vi "New plot1_old.vi"() -> (0 "Closed w":bool)   [LabVIEW 2021]
uses:
  <vilib>/Analysis/NI_AALBase.lvlib
  <vilib>/gmath/NI_Gmath.lvlib
  <vilib>/Analysis/1siggen.llb/Ramp Pattern by Samples.vi
panel:
  in  "Tab Control":enum32{"Graph", "Information"}(tab)
  out "Waveform Graph":waveform(dbl)[](graph) caption="Waveform Graph 2"
  in  "Local Mode":enum32{"Resume", "Hold"}(radio)
  in  "Refresh time":u32
  out "Filename":string
  out "Trace name":string
  out "Mode signal_Global":string
  out "Execution:State":T1(ring)
  out "total \nrefresh time":u32
  out "message":string
  in  "Minimizar":bool
  in  "stop":bool
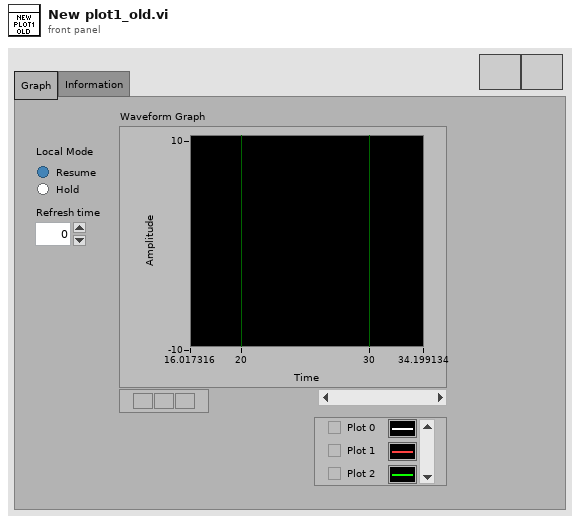
[diagram p1: front panel]
types:
  T1 = enum32{"Bad", "Idle", "Run top level", "Running"}
  T2 = cluster{"plot Names":string[], "Waveforms arrays":waveform(dbl)[], "signals_HW":string[][], "Waveforms arrays csv":waveform(dbl)[], "signals_csv":string[], "Signals_name":string[], "Mode_signal_conf":u8, "Request_plots_array":cluster{string, waveform(dbl)}[], "time out":i32, " global r time":u32}
  T3 = enum32{"Invalid", "Standard", "Closed", "Hidden", "Minimized", "Maximized"}
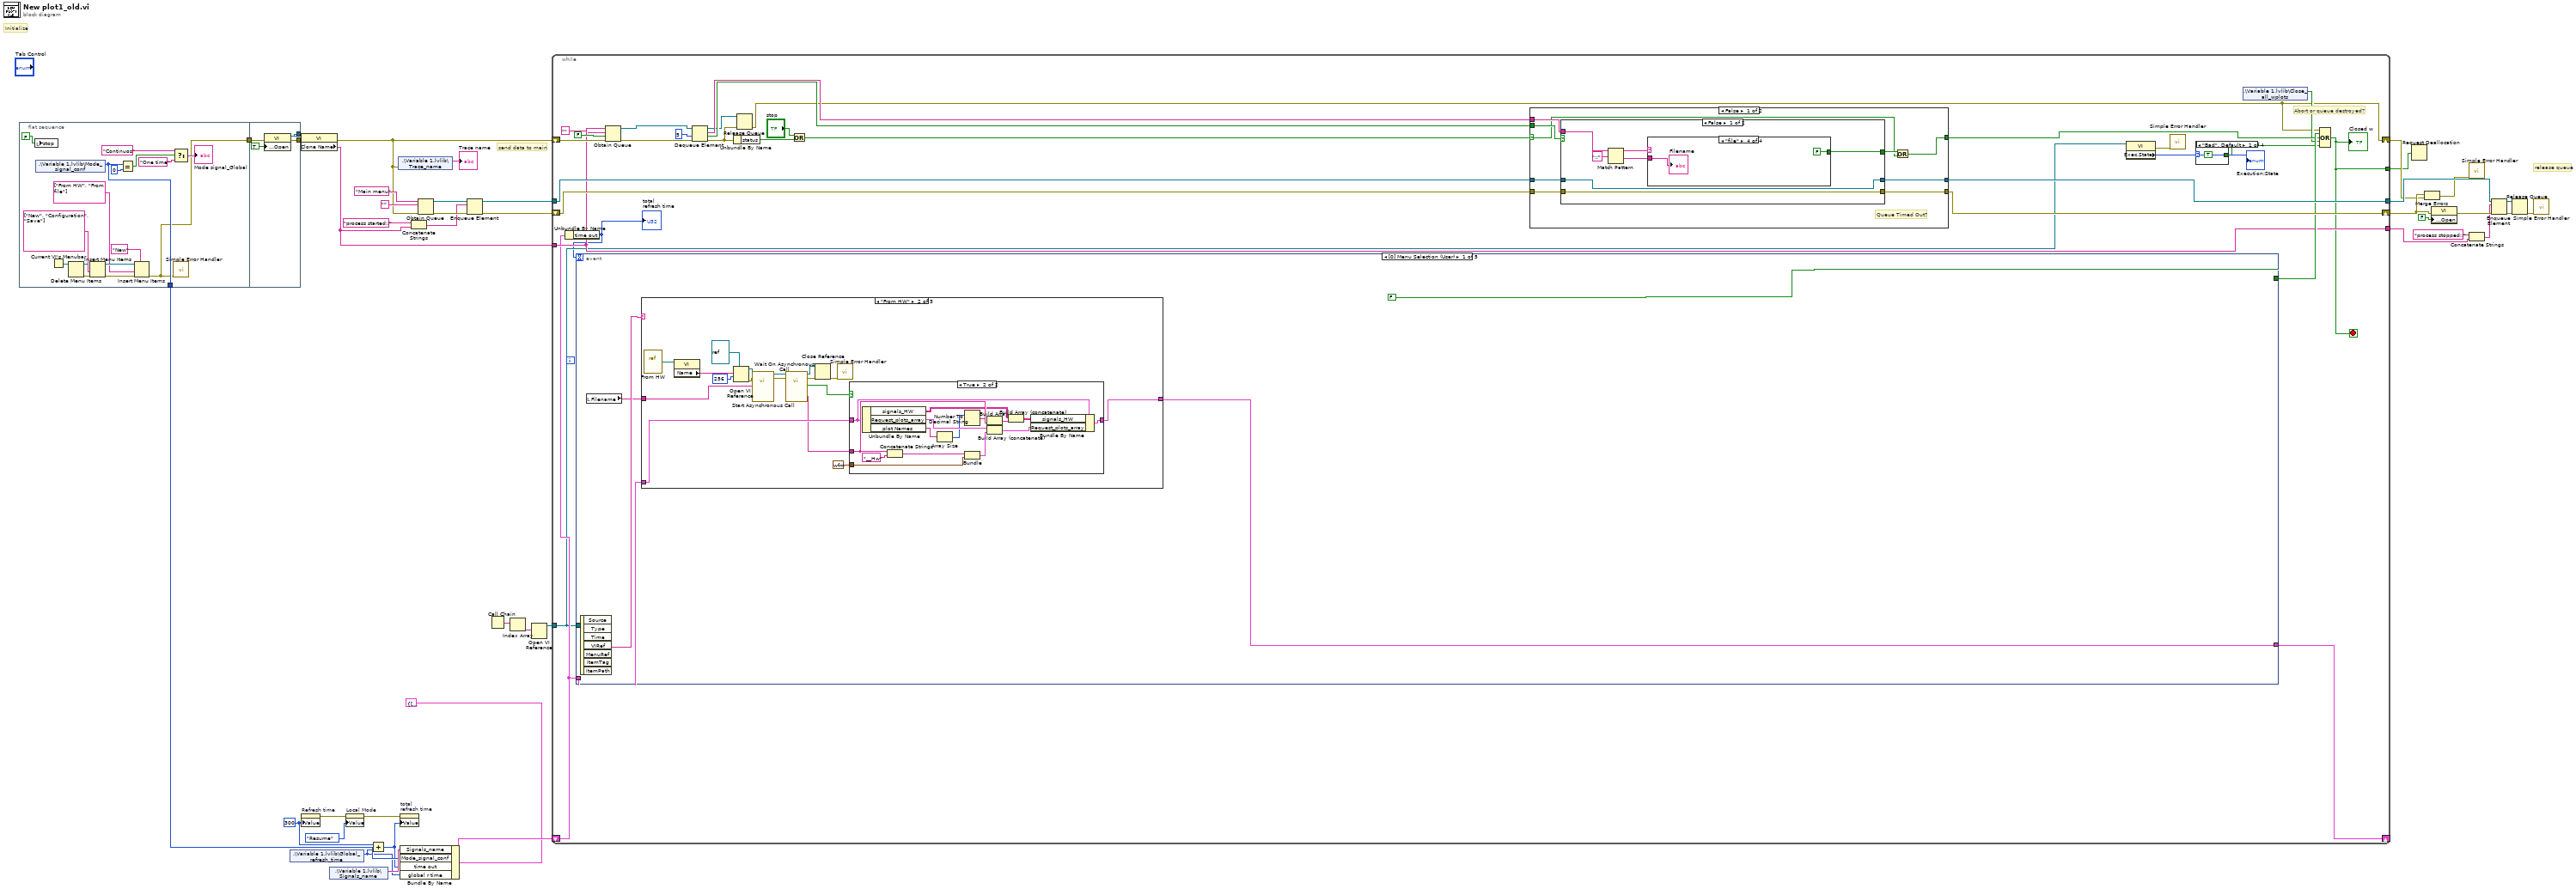
[diagram p0: block diagram]
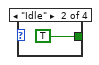
[diagram p2: hidden frame]
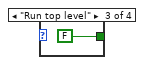
[diagram p3: hidden frame]
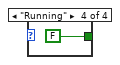
[diagram p4: hidden frame]
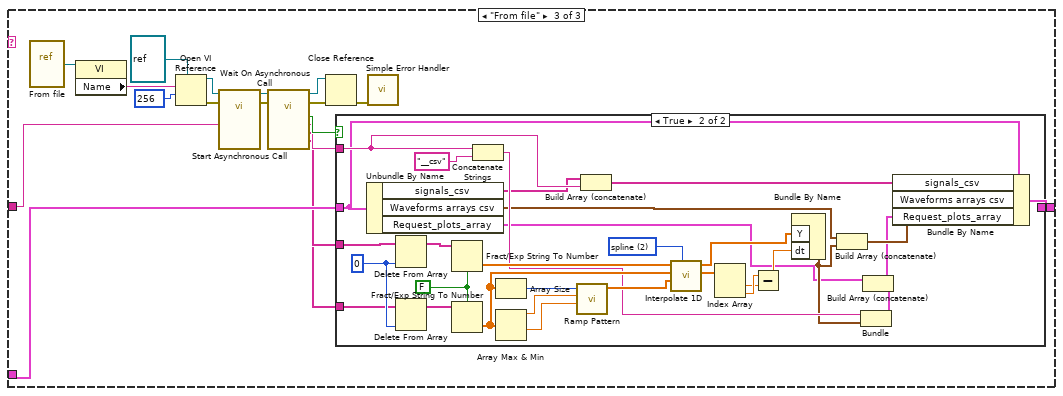
[diagram p7: hidden frame]
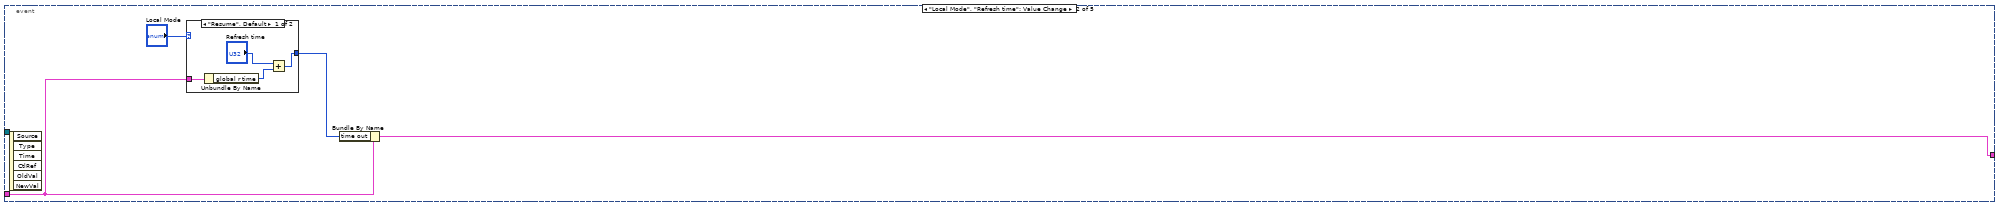
[diagram p9: hidden frame]
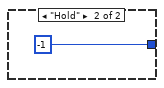
[diagram p10: hidden frame]
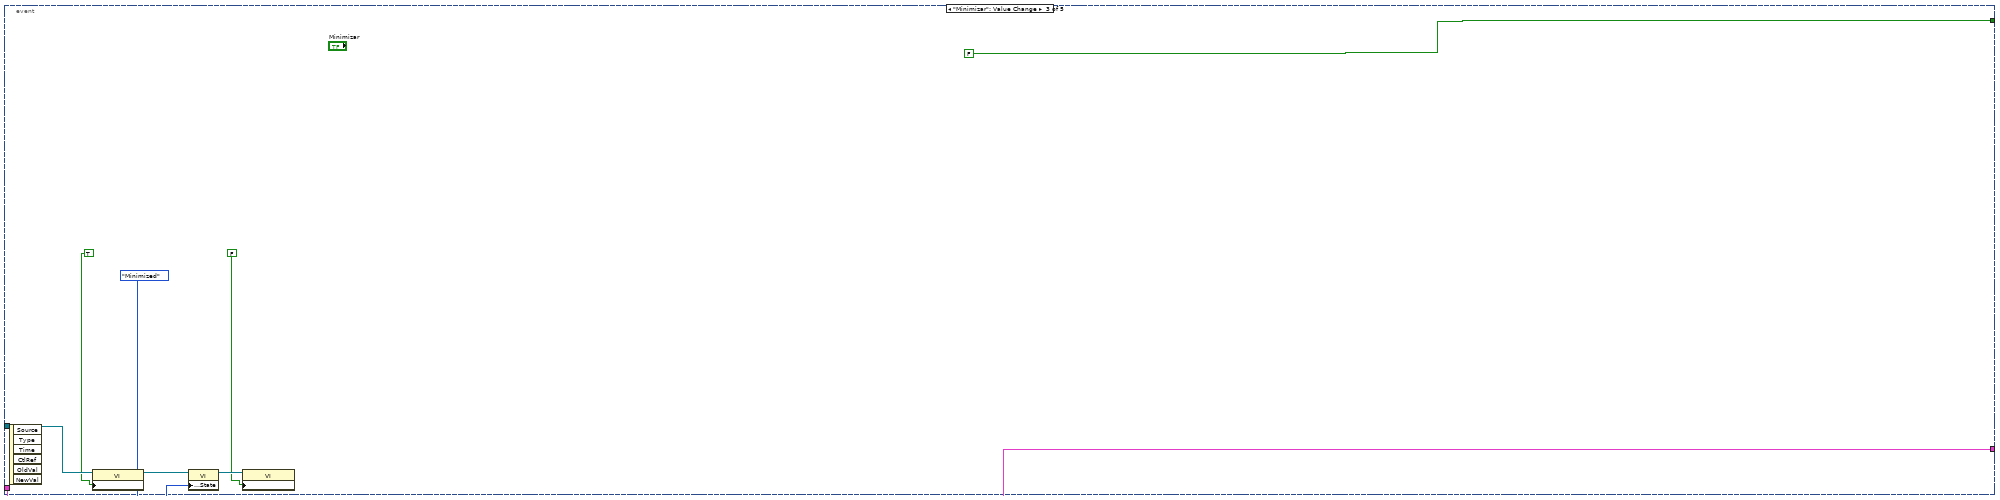
[diagram p11: hidden frame]
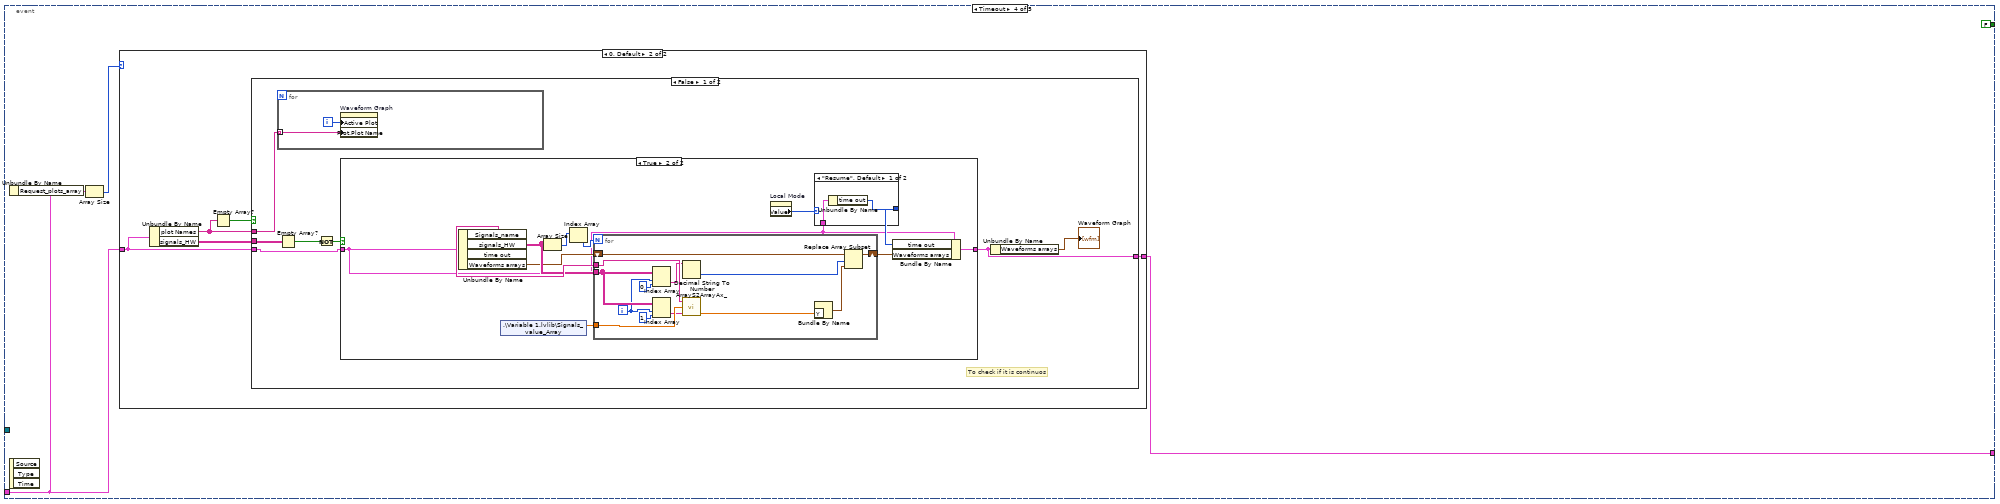
[diagram p12: hidden frame]
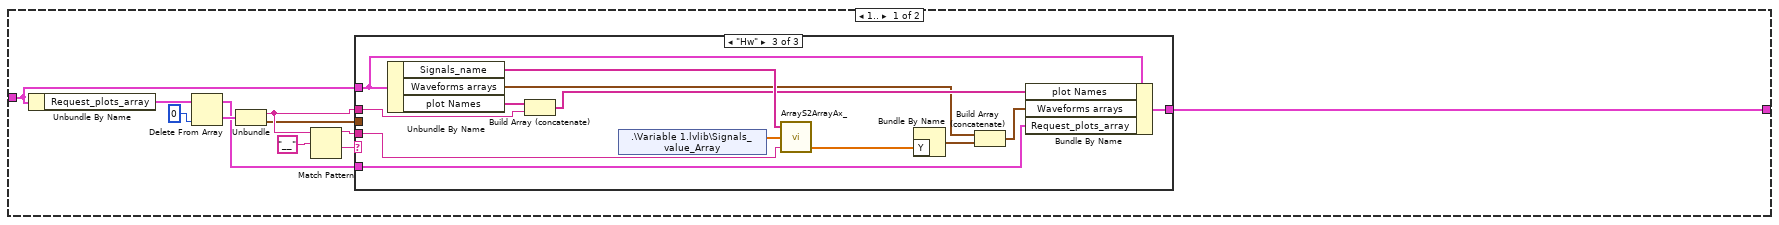
[diagram p13: hidden frame]
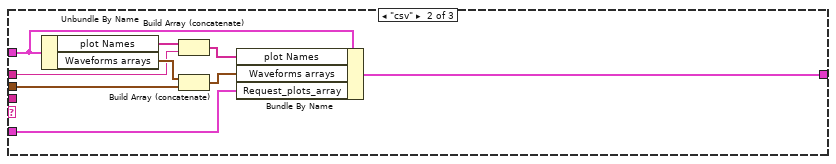
[diagram p15: hidden frame]
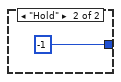
[diagram p17: hidden frame]
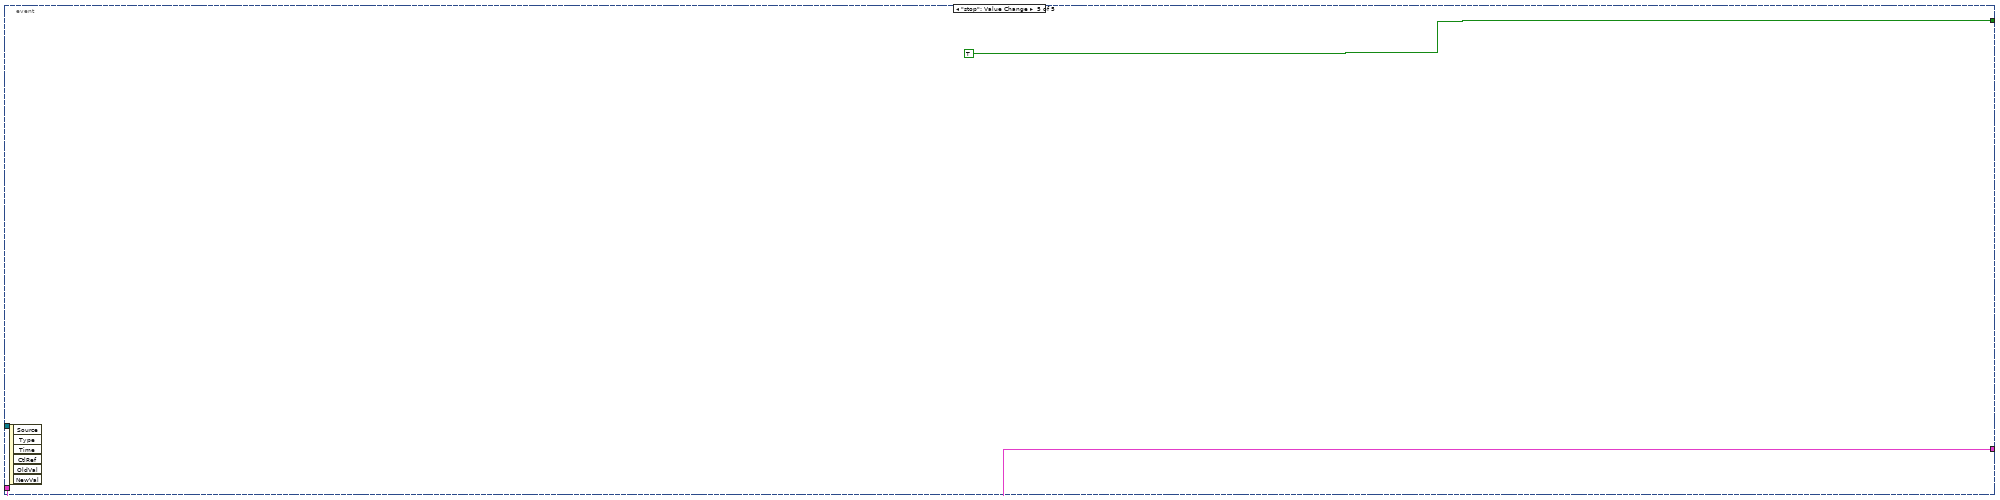
[diagram p19: hidden frame]
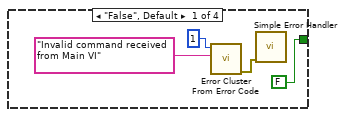
[diagram p20: hidden frame]
diagram:
  w5 = u32 300 ("Refresh time")
  # "Initialize"
  # "send data to main"
  # "release queue"
  n1 = flat-sequence {
    tunnel: [w42] -> w12
    tunnel: [w41] -> w1
    tunnel: [w59] -> w19
    tunnel: [w58] -> w34
    tunnel: w1 -> [w57]
    frame #0 {
      n2 = local write "stop"(FALSE ("stop")) -> ()
      n3 = shared-variable ".\\Variable 1.lvlib\\Mode_signal_conf"() -> (w42:u8)  [unwired: 1 in, 1 out]
      n4 = Current VI's Menubar() -> (w51:refnum<k9>)
      n5 = Delete Menu Items(9:w51) -> (0:w50:errorcluster, 3:w49:refnum<k9>)  [unwired: 3 in]
      n6 = Insert Menu Items(6:w50, 7:string[] ["New", "Configuration", "Save"], 9:w49) -> (0:w56:errorcluster, 3:w55:refnum<k9>)  [unwired: 3 in, 1 out]
      n7 = Equal?(x=w42, y=u8 0) -> (x = y?=w46:bool)
      n8 = Insert Menu Items(5:"New", 6:w56, 7:string[] ["From HW", "From file"], 9:w55) -> (0:w41:errorcluster)  [unwired: 2 in, 2 out]
      n9 = Select(t="Continuos", s=w46, f="One time") -> (s? t:f=→"Mode signal_Global":string)
      n10 = call <vilib>:"Simple Error Handler.vi"("error in (no error)"=w41) -> ()  [unwired: 4 in, 5 out]
    }
    frame #1 {
      n11 = property class="VI"(error in=w57, "Front Panel.Open"=TRUE ("Front Panel Window:Open")) -> (reference out=w59:refnum<vi>, error out=w58:errorcluster)  [unwired: 1 in]
    }
  }
  n12 = shared-variable ".\\Variable 1.lvlib\\Global_refresh_time"() -> (w2:u16)  [unwired: 1 in, 1 out]
  n13 = property class="VI"(reference=w19, error in=w34) -> (error out=w10:errorcluster, "Clone Name"=w11:string)  [unwired: 1 out]
  n14 = property on="Refresh time" class="DigNum (strict)"("Value"=w5) -> (error out=w8:errorcluster)  [unwired: 2 in, 1 out]
  n15 = shared-variable ".\\Variable 1.lvlib\\Signals_name"() -> (w13:string[])  [unwired: 1 in, 1 out]
  n16 = property on="Local Mode" class="RadioBtnsControl (strict)"(error in=w8, "Value"=enum32{"Resume", "Hold"}."Resume" ("Local Mode")) -> (error out=w4:errorcluster)  [unwired: 1 in, 1 out]
  n17 = Add(x=w5, y=w2) -> (x+y=w3:u32)
  n18 = shared-variable ".\\Variable 1.lvlib\\Trace_name"(error in=w10) -> (→"Trace name":string)  [unwired: 1 out]
  n19 = property on="total \nrefresh time" class="DigNum (strict)"(error in=w4, "Value"=w3) -> ()  [unwired: 1 in, 2 out]
  n20 = Bundle By Name(cluster=T2 {"plot Names"=[], "Waveforms arrays"=[], "signals_HW"=[], "Waveforms arrays csv"=[], "signals_csv"=[], "Signals_name"=[], "Mode_signal_conf"=0, "Request_plots_array"=[], "time out"=300, " global r time"=0}, "Signals_name"=w13, "Mode_signal_conf"=w12, "time out"=w3, "global r time"=w2) -> (w14:T2)
  n21 = Concatenate Strings("process started::" ("name (unnamed)"), w11) -> (w35:string)
  n22 = Obtain Queue(name (unnamed)="Main menu", element data type="", error in (no error)=w10) -> (queue out=w37:refnum<queue>, error out=w36:errorcluster)  [unwired: 2 in, 1 out]
  n23 = Enqueue Element(queue=w37, element=w35, error in (no error)=w36) -> (queue out=w33:refnum<queue>, error out=w32:errorcluster)  [unwired: 1 in, 1 out]
  n24 = Call Chain() -> (call chain=w18:string[])
  n25 = Index Array(array=w18) -> (element=w17:string)  [unwired: 1 in]
  n26 = Open VI Reference(vi path=w17) -> (vi reference=w16:refnum<vi>)  [unwired: 5 in, 1 out]
  n27 = while {
    tunnel: w33 -> [w90]
    tunnel: [w88] -> w31
    shift-right: [w87] -> w25
    shift-left: w32 -> [w89]
    shift-right: [w61] -> w24
    shift-left: w10 -> [w78]
    tunnel: [w70] -> w21
    tunnel: w16 -> [w66]
    tunnel: w11 -> [w70]
    shift-right: [w71] -> _
    shift-left: w14 -> [w69]
    tunnel: [w63] -> w7
    stop <- w63 stop-if-true
    # "Abort or queue destroyed?"
    n28 = Unbundle By Name(w69) -> ("time out"=w62:i32)
    "total \nrefresh time" <- w62
    n29 = event shown="[0] Menu Selection (User)" {
      selector: _ -> [_ _ _ _ _]
      dyn-events: _ -> [_ _ _ _ _]
      timeout: w62 -> [_ _ _ _ _]
      tunnel: [FALSE _ FALSE FALSE TRUE] -> w74
      tunnel: w66 -> [_ _ w199 _ _]
      tunnel: [w96 w186 w193 w204 w283] -> w71
      tunnel: w69 -> [w97 w184 w193 w203 w283]
      event Menu Selection (User) {
        n30 = event-data() -> ("ItemTag"=w99:string)  [unwired: 1 in, 6 out]
        n31 = local read "Filename"() -> (w95:string)
        n32 = case shown="\"From HW\"" w99 {
          tunnel: [w100 w112 w144] -> w96
          tunnel: w97 -> [w100 w103 w145]
          tunnel: w95 -> [_ w104 w134]
          frame "False", Default {
          }
          frame "From HW" {
            n33 = vi-ref "From HW.vi"() -> (w113:refnum<vi>)
            n34 = property class="VI"(reference=w113) -> ("Name"=w105:string)  [unwired: 1 in, 2 out]
            n35 = Open VI Reference(type specifier VI Refnum (for type only)=refnum<vi> refnum ("reference"), vi path=w105, options=256) -> (vi reference=w114:refnum<vi>, error out=w117:errorcluster)  [unwired: 3 in]
            n36 = call-by-ref "Start Asynchronous Call"(reference=w114, error in=w117, "Plot window"=w104) -> (reference out=w110:refnum<vi>, error out=w111:errorcluster)  [unwired: 2 in, 3 out]
            n37 = call-by-ref "Wait On Asynchronous Call"(reference=w110, error in=w111) -> (reference out=w109:refnum<vi>, error out=w108:errorcluster, "Y name"=w101:string, "Ready?"=w107:bool)  [unwired: 3 in, 1 out]
            n38 = Close Reference(reference=w109, error in (no error)=w108) -> (error out=w116:errorcluster)
            n39 = call <vilib>:"Simple Error Handler.vi"("error in (no error)"=w116) -> ()  [unwired: 4 in, 5 out]
            n40 = case shown="True" w107 {
              tunnel: w101 -> [_ w132]
              tunnel: [w118 w127] -> w112
              tunnel: w103 -> [w118 w131]
              tunnel: waveform(dbl) {"t0"=timestamp(0 s since 1904-01-01), "dt"=1.0, "Y"=[]} ("Waveform") -> [_ w125]
              frame False {
              }
              frame True {
                n41 = Unbundle By Name(w131) -> ("signals_HW"=w130:string[][], "Request_plots_array"=w124:cluster{string, waveform(dbl)}[], "plot Names"=w121:string[])
                n42 = Concatenate Strings(w132, "__Hw" ("string")) -> (w126:string)
                n43 = Array Size(array=w121) -> (size(s)=w120:i32)
                n44 = Number To Decimal String(number=w120) -> (decimal integer string=w119:string)  [unwired: 1 in]
                n45 = Bundle(w126, "Waveform"=w125) -> (w123:cluster{string, "Waveform":waveform(dbl)})  [unwired: 1 in]
                n46 = Build Array(w119, w132) -> (w129:string[])
                n47 = Build Array (concatenate)(w124, w123) -> (w122:cluster{string, "Waveform":waveform(dbl)}[])
                n48 = Build Array (concatenate)(w130, w129) -> (w128:string[][])
                n49 = Bundle By Name(cluster=w131, "signals_HW"=w128, "Request_plots_array"=w122) -> (w127:T2)
              }
            }
          }
          frame "From file" {
            n50 = vi-ref "From file.vi"() -> (w148:refnum<vi>)
            n51 = property class="VI"(reference=w148) -> ("Name"=w142:string)  [unwired: 1 in, 2 out]
            n52 = Open VI Reference(type specifier VI Refnum (for type only)=refnum<vi> refnum, vi path=w142, options=256) -> (vi reference=w146:refnum<vi>, error out=w151:errorcluster)  [unwired: 3 in]
            n53 = call-by-ref "Start Asynchronous Call"(reference=w146, error in=w151, "Plot window"=w134) -> (reference out=w143:refnum<vi>, error out=w141:errorcluster)  [unwired: 3 in, 4 out]
            n54 = call-by-ref "Wait On Asynchronous Call"(reference=w143, error in=w141) -> (reference out=w136:refnum<vi>, error out=w135:errorcluster, "Y subarray"=w137:string[], "X subarray"=w138:string[], "Curve name"=w139:string, "Ready?"=w140:bool)  [unwired: 4 in]
            n55 = Close Reference(reference=w136, error in (no error)=w135) -> (error out=w150:errorcluster)
            n56 = case shown="True" w140 {
              tunnel: w138 -> [_ w182]
              tunnel: w137 -> [_ w181]
              tunnel: w139 -> [_ w164]
              tunnel: w145 -> [w152 w158]
              tunnel: [w152 w159] -> w144
              frame False {
              }
              frame True {
                w173 = 2 items=["nearest", "linear", "spline", "cubic Hermite", "Lagrange"] ("method")
                w178 = FALSE ("use system decimal point (T)")
                w183 = 0 ("index")
                n57 = Unbundle By Name(w158) -> ("signals_csv"=w156:string[], "Waveforms arrays csv"=w157:waveform(dbl)[], "Request_plots_array"=w155:cluster{string, waveform(dbl)}[])
                n58 = Delete From Array(array=w182, index=w183) -> (array with subset deleted=w179:string[])  [unwired: 1 in, 1 out]
                n59 = Delete From Array(array=w181, index=w183) -> (array with subset deleted=w180:string[])  [unwired: 1 in, 1 out]
                n60 = Fract/Exp String To Number(use system decimal point (T)=w178, string=w179) -> (number=w170:dbl[])  [unwired: 2 in, 1 out]
                n61 = Fract/Exp String To Number(use system decimal point (T)=w178, string=w180) -> (number=w172:dbl[])  [unwired: 2 in, 1 out]
                n62 = Concatenate Strings(w164, "__csv" ("string")) -> (w163:string)
                n63 = Array Size(array=w172) -> (size(s)=w176:i32)
                n64 = Array Max & Min(array=w172) -> (max value=w175:dbl, min value=w174:dbl)  [unwired: 2 out]
                n65 = call-poly <vilib>:"Ramp Pattern.vi"("start"=w174, "end"=w175, "samples"=w176) -> ("Ramp Pattern"=w171:dbl[])  [unwired: 7 in, 1 out]
                n66 = Build Array (concatenate)(w156, w164) -> (w161:string[])
                n67 = call <vilib>:"Interpolate 1D.vi"("method"=w173, "xi"=w171, "X"=w172, "Y"=w170) -> ("xi used"=w169:dbl[], "yi"=w168:dbl[])  [unwired: 5 in, 1 out]
                n68 = Index Array(array=w169) -> (element #1=w166:dbl, element #2=w167:dbl)  [unwired: 2 in]
                n69 = Subtract(x=w167, y=w166) -> (x-y=w165:dbl)
                n70 = Bundle By Name("Y"=w168, "dt"=w165) -> (w162:waveform(dbl))  [unwired: 1 in]
                n71 = Build Array (concatenate)(w157, w162) -> (w160:waveform(dbl)[])
                n72 = Bundle(w163, w162) -> (w154:cluster{string, waveform(dbl)})  [unwired: 1 in]
                n73 = Build Array (concatenate)(w155, w154) -> (w153:cluster{string, waveform(dbl)}[])
                n74 = Bundle By Name(cluster=w158, "signals_csv"=w161, "Waveforms arrays csv"=w160, "Request_plots_array"=w153) -> (w159:T2)
              }
            }
            n75 = call <vilib>:"Simple Error Handler.vi"("error in (no error)"=w150) -> ()  [unwired: 4 in, 5 out]
          }
        }
      }
      event "Local Mode", "Refresh time": Value Change {
        n76 = event-data() -> ()  [unwired: 1 in, 6 out]
        n77 = case shown="\"Resume\", Default" "Local Mode" {
          tunnel: [w188 -1 ("time out")] -> w187
          tunnel: w184 -> [w191 _]
          frame "Resume", Default {
            n78 = Unbundle By Name(w191) -> ("global r time"=w189:u32)
            n79 = Add(x="Refresh time", y=w189) -> (x+y=w188:u32)
          }
          frame "Hold" {
          }
        }
        n80 = Bundle By Name(cluster=w184, "time out"=w187) -> (w186:T2)
      }
      event "Minimizar": Value Change {
        n81 = event-data() -> ()  [unwired: 1 in, 6 out]
        n82 = property class="VI"(reference=w199, "Front Panel.Minimizeable"=TRUE ("Front Panel Window:Minimizable")) -> (reference out=w198:refnum<vi>)  [unwired: 1 in, 1 out]
        n83 = property class="VI"(reference=w198, "Front Panel Window:State"=T3."Minimized") -> (reference out=w196:refnum<vi>)  [unwired: 1 in, 1 out]
        n84 = property class="VI"(reference=w196, "Front Panel.Minimizeable"=FALSE ("Front Panel Window:Minimizable")) -> ()  [unwired: 1 in, 2 out]
      }
      event Timeout {
        n85 = Unbundle By Name(w203) -> ("Request_plots_array"=w202:cluster{string, waveform(dbl)}[])
        n86 = event-data() -> ()  [unwired: 1 in, 3 out]
        n87 = Array Size(array=w202) -> (size(s)=w201:i32)
        n88 = case shown="0, Default" w201 {
          tunnel: w203 -> [w212 w242]
          tunnel: [w213 w241] -> w204
          frame 1.. {
            n89 = Unbundle By Name(w212) -> ("Request_plots_array"=w207:cluster{string, waveform(dbl)}[])
            n90 = Delete From Array(array=w207, index=0) -> (deleted portion=w208:cluster{string, waveform(dbl)}, array with subset deleted=w206:cluster{string, waveform(dbl)}[])  [unwired: 1 in]
            n91 = Unbundle(w208) -> (w210:string, w209:waveform(dbl))
            n92 = Match Pattern(string=w210, regular expression="__") -> (before substring=w214:string, after substring=w215:string)  [unwired: 1 in, 2 out]
            n93 = case shown="\"Hw\"" w215 {
              tunnel: w212 -> [w217 w226 w235]
              tunnel: w214 -> [_ _ w237]
              tunnel: w209 -> [_ w223 _]
              tunnel: w210 -> [_ w221 w234]
              tunnel: [w217 w219 w230] -> w213
              tunnel: w206 -> [_ w218 w228]
              frame "False", Default {
              }
              frame "csv" {
                n94 = Unbundle By Name(w226) -> ("plot Names"=w225:string[], "Waveforms arrays"=w224:waveform(dbl)[])
                n95 = Build Array (concatenate)(w225, w221) -> (w220:string[])
                n96 = Build Array (concatenate)(w224, w223) -> (w222:waveform(dbl)[])
                n97 = Bundle By Name(cluster=w226, "plot Names"=w220, "Waveforms arrays"=w222, "Request_plots_array"=w218) -> (w219:T2)
              }
              frame "Hw" {
                n98 = Unbundle By Name(w235) -> ("Signals_name"=w238:string[], "Waveforms arrays"=w227:waveform(dbl)[], "plot Names"=w229:string[])
                n99 = Build Array (concatenate)(w229, w234) -> (w233:string[])
                n100 = shared-variable ".\\Variable 1.lvlib\\Signals_value_Array"() -> (w239:dbl[])  [unwired: 1 in, 1 out]
                n101 = call "ArrayS2ArrayAx_.vi"("Signal_input"=w237, "Signals_value_Array"=w239, "Signals_name"=w238) -> ("Subarray 1x_out"=w236:sgl[])  [unwired: 2 out]
                n102 = Bundle By Name("Y"=w236) -> (w232:waveform(sgl))  [unwired: 1 in]
                n103 = Build Array (concatenate)(w227, w232) -> (w231:waveform(dbl)[])
                n104 = Bundle By Name(cluster=w235, "plot Names"=w233, "Waveforms arrays"=w231, "Request_plots_array"=w228) -> (w230:T2)
              }
            }
          }
          frame 0, Default {
            n105 = Unbundle By Name(w242) -> ("plot Names"=w244:string[], "signals_HW"=w240:string[][])
            n106 = Empty Array?(array=w244) -> (empty?=w243:bool)
            n107 = case shown="False" w243 {
              tunnel: w244 -> [w251 _]
              tunnel: w240 -> [w249 _]
              tunnel: w242 -> [w250 w282]
              tunnel: [w245 w282] -> w241
              frame False {
                # "To check if it is continuos"
                n108 = for {
                  tunnel: w251 -> [w280] mode=indexing
                  i -> [w281]
                  n109 = property on="Waveform Graph" class="WFGraph (strict)"("Active Plot"=w281, "Plot.Plot Name"=w280) -> ()  [unwired: 2 in, 2 out]
                }
                n110 = Empty Array?(array=w249) -> (empty?=w248:bool)
                n111 = Not(x=w248) -> (.not. x?=w247:bool)
                n112 = case shown="True" w247 {
                  tunnel: w250 -> [w252 w253]
                  tunnel: [w252 w257] -> w245
                  frame False {
                  }
                  frame True {
                    n113 = Unbundle By Name(w253) -> ("Signals_name"=w262:string[], "signals_HW"=w261:string[][], "Waveforms arrays"=w258:waveform(dbl)[])  [unwired: 1 out]
                    n114 = shared-variable ".\\Variable 1.lvlib\\Signals_value_Array"() -> (w263:dbl[])  [unwired: 1 in, 1 out]
                    n115 = Array Size(array=w261) -> (size(s)=w260:i32[])
                    n116 = Index Array(array=w260) -> (element=w259:i32)  [unwired: 1 in]
                    n117 = for {
                      N: w259 -> [_]
                      tunnel: w261 -> [w277]
                      tunnel: w263 -> [w279]
                      tunnel: w262 -> [w278]
                      shift-right: [w267] -> w254
                      shift-left: w258 -> [w272]
                      i -> [w269]
                      n118 = Index Array(array=w277, index (row)=w269, index (col)=0 ("disabled index (row)")) -> (element=w275:string)
                      n119 = Index Array(array=w277, index (row)=w269, index (col)=1 ("index")) -> (element=w276:string)
                      n120 = Decimal String To Number(string=w275) -> (number=w271:i32)  [unwired: 2 in, 1 out]
                      n121 = call "ArrayS2ArrayAx_.vi"("Signal_input"=w276, "Signals_value_Array"=w279, "Signals_name"=w278) -> ("Subarray 1x_out"=w274:sgl[])  [unwired: 2 out]
                      n122 = Bundle By Name("Y"=w274) -> (w273:waveform(sgl))  [unwired: 1 in]
                      n123 = Replace Array Subset(array=w272, new element=w273, index=w271) -> (w267:waveform(dbl)[])
                    }
                    n124 = property on="Local Mode" class="RadioBtnsControl (strict)"() -> ("Value"=w256:enum32{"Resume", "Hold"})  [unwired: 2 in, 2 out]
                    n125 = case shown="\"Resume\", Default" w256 {
                      tunnel: [w264 -1 ("time out")] -> w255
                      tunnel: w253 -> [w265 _]
                      frame "Resume", Default {
                        n126 = Unbundle By Name(w265) -> ("time out"=w264:i32)
                      }
                      frame "Hold" {
                      }
                    }
                    n127 = Bundle By Name(cluster=w253, "time out"=w255, "Waveforms arrays"=w254) -> (w257:T2)
                  }
                }
                n128 = Unbundle By Name(w245) -> ("Waveforms arrays"=→"Waveform Graph":waveform(dbl)[])
              }
              frame True {
              }
            }
          }
        }
      }
      event "stop": Value Change {
        n129 = event-data() -> ()  [unwired: 1 in, 6 out]
      }
    }
    n130 = Obtain Queue(name (unnamed)=w70, element data type="", create if not found? (T)=FALSE, error in (no error)=w78) -> (queue out=w80:refnum<queue>, error out=w79:errorcluster)  [unwired: 1 in, 1 out]
    n131 = Dequeue Element(queue=w80, timeout in ms (-1)=5, error in (no error)=w79) -> (queue out=w76:refnum<queue>, element=w83:string, timed out?=w84:bool, error out=w75:errorcluster)
    n132 = Unbundle By Name(w75) -> ("status"=w82:bool)
    n133 = Release Queue(queue=w76, error in (no error)=w75) -> (error out=w61:errorcluster)  [unwired: 1 in, 2 out]
    n134 = Or(x="stop", y=w82) -> (x .or. y?=w81:bool)
    n135 = case shown="False" w81 {
      selector: w81 -> [w290 w317]
      tunnel: [w289 w317] -> w73
      tunnel: w90 -> [w286 w316]
      tunnel: w89 -> [w288 w315]
      tunnel: [w285 w316] -> w88
      tunnel: [w287 w315] -> w87
      tunnel: w84 -> [w293 _]
      tunnel: w83 -> [w292 _]
      frame False {
        # "Queue Timed Out?"
        n136 = case shown="False" w293 {
          tunnel: w292 -> [w299 _]
          tunnel: [w297 FALSE] -> w291
          tunnel: w288 -> [w296 w314]
          tunnel: [w296 w314] -> w287
          tunnel: w286 -> [w295 w313]
          tunnel: [w295 w313] -> w285
          frame False {
            n137 = Match Pattern(string=w299, regular expression="::") -> (before substring=w300:string, after substring=w294:string)  [unwired: 1 in, 2 out]
            n138 = case shown="\"file\"" w300 {
              tunnel: [FALSE TRUE w306 FALSE] -> w297
              tunnel: w294 -> [_ _ w307 w309]
              frame "False", Default {
                n139 = call <vilib>:"Error Cluster From Error Code.vi"("error message (\"\")"="Invalid command received from Main VI" ("error message (\"\")"), "error code (0)"=1) -> ("error out"=w302:errorcluster)  [unwired: 7 in]
                n140 = call <vilib>:"Simple Error Handler.vi"("error in (no error)"=w302) -> ()  [unwired: 4 in, 5 out]
              }
              frame "exit" {
              }
              frame "message" {
                n141 = Equal?(x=w307, y="stop") -> (x = y?=w306:bool)
                "message" <- w307
              }
              frame "file" {
                "Filename" <- w309
              }
            }
          }
          frame True {
            n142 = Wait (ms)(milliseconds to wait=u32 10) -> ()  [unwired: 1 out]
          }
        }
        n143 = Or(x=w291, y=w290) -> (x .or. y?=w289:bool)
      }
      frame True {
      }
    }
    n144 = property class="VI"(reference=w66) -> (error out=w65:errorcluster, "Exec.State"=w68:T1)  [unwired: 1 in, 1 out]
    "Execution:State" <- w68
    n145 = call <vilib>:"Simple Error Handler.vi"("error in (no error)"=w65) -> ()  [unwired: 4 in, 5 out]
    n146 = case shown="\"Bad\", Default" w68 {
      tunnel: [TRUE ("value") TRUE ("value") FALSE ("value") FALSE ("value")] -> w67
      frame "Bad", Default {
      }
      frame "Idle" {
      }
      frame "Run top level" {
      }
      frame "Running" {
      }
    }
    n147 = shared-variable ".\\Variable 1.lvlib\\Close_all_wplots"() -> (w72:bool)  [unwired: 1 in, 1 out]
    n148 = Compound Arithmetic op=OR(w61, w74, w73, w72, w67) -> (w63:bool)
    "Closed w" <- w63
  }
  n149 = Request Deallocation(w7) -> ()
  n150 = Merge Errors(w25, w24) -> (w15:errorcluster)
  n151 = property class="VI"(error in=w25, "Front Panel.Open"=FALSE ("Front Panel Window:Open")) -> (error out=w27:errorcluster)  [unwired: 1 in, 1 out]
  n152 = call <vilib>:"Simple Error Handler.vi"("error in (no error)"=w15) -> ()  [unwired: 4 in, 5 out]
  n153 = Concatenate Strings("process stopped::" ("string"), w21) -> (w20:string)
  n154 = Enqueue Element(queue=w31, element=w20, error in (no error)=w27) -> (queue out=w30:refnum<queue>, error out=w29:errorcluster)  [unwired: 1 in, 1 out]
  n155 = Release Queue(queue=w30, error in (no error)=w29) -> (error out=w28:errorcluster)  [unwired: 1 in, 2 out]
  n156 = call <vilib>:"Simple Error Handler.vi"("error in (no error)"=w28) -> ()  [unwired: 4 in, 5 out]
